vi "字符串连接.vi"() -> ()   [LabVIEW 2018]
panel:
  out "字符串":string
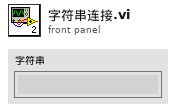
[diagram p1: front panel]
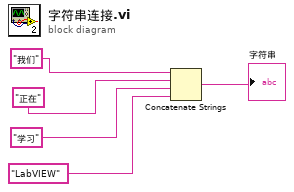
[diagram p0: block diagram]
diagram:
  n1 = Concatenate Strings("我们", "正在", "学习", "LabVIEW") -> (→"字符串":string)
